vi "StageInit.vi"(1 "error in (no error)":errorcluster) -> (0 "error out":errorcluster)   [LabVIEW 2009]
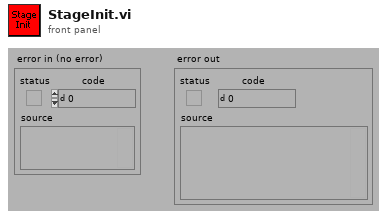
[diagram p1: front panel]
types:
  T1 = enum16{"Get Type", "Set Type", "GetStageInit", "GetWriteStageSetting", "GetInitializeStageOutput", "GetSetAxisPosition", "GetSetPos"}
  T2 = typedef "StageType.ctt" = enum16{"PI analogue", "PI 712 TCP/IP", "Märzhäuser", "PI analogue step", "PI 712 USB"}
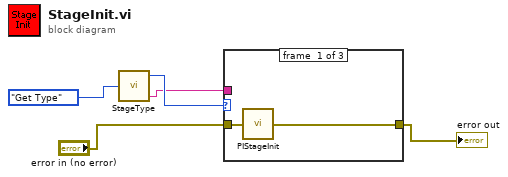
[diagram p0: block diagram]
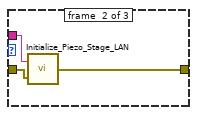
[diagram p2: hidden frame]
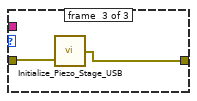
[diagram p3: hidden frame]
diagram:
  n1 = call "StageType.vi"("Function"=T1."Get Type") -> ("Host address (out)"=w1:string, "Stage Type (output)"=w2:T2)  [unwired: 2 in, 1 out]
  n2 = case shown="\"PI 712 USB\"" w2 {
    tunnel: "error in (no error)" -> [w7 w10 w12]
    tunnel: [w6 w9 w11] -> w4
    tunnel: w1 -> [_ w8 _]
    frame #0 {
      n3 = call "PIStageInit.vi"("error in (no error)"=w7) -> ("error out"=w6:errorcluster)
    }
    frame #1 {
      n4 = call "Initialize_Piezo_Stage_LAN.vi"("error in"=w10, "Host address/name"=w8) -> ("error out"=w9:errorcluster)
    }
    frame #2 {
      n5 = call "Initialize_Piezo_Stage_USB.vi"("error in"=w12) -> ("error out"=w11:errorcluster)  [unwired: 1 in]
    }
  }
  "error out" <- w4
